vi "INTERFAZ.vi"() -> ()   [LabVIEW 2020]
panel:
  in  "Modo Nocturno":bool
  in  "stop":bool
  in  "Tab Control":enum32{"Page 1", "Page 2"}(tab)
  out "Contraseña":bool
  out "Usuario":bool
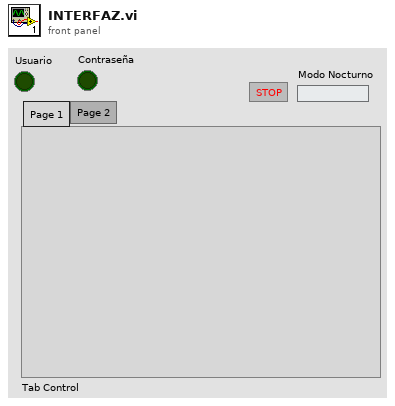
[diagram p1: front panel]
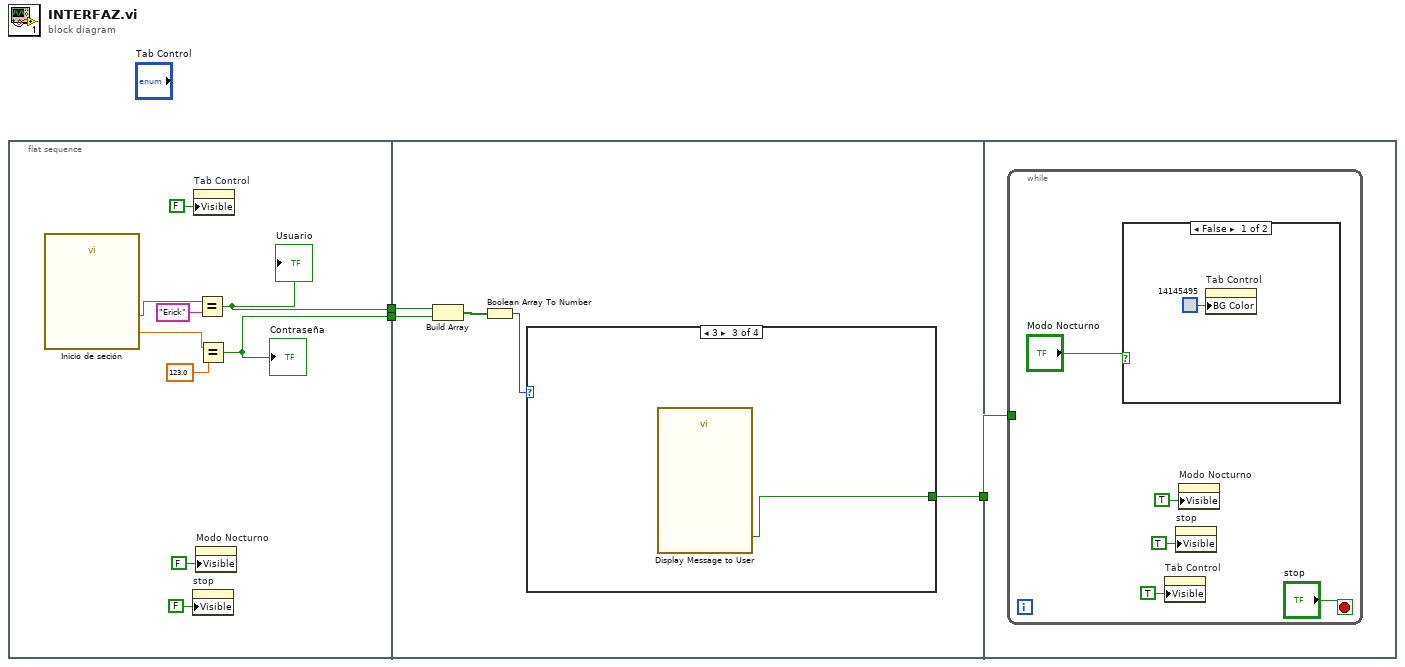
[diagram p0: block diagram]
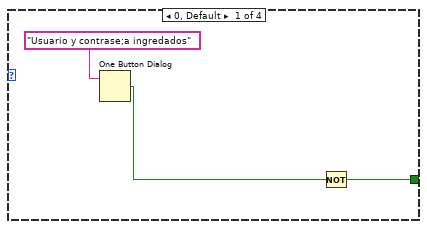
[diagram p2: hidden frame]
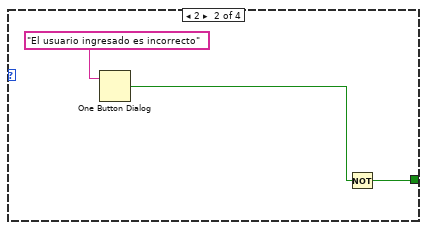
[diagram p3: hidden frame]
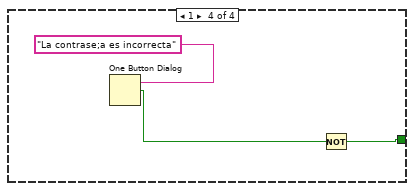
[diagram p4: hidden frame]
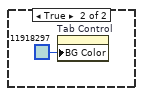
[diagram p5: hidden frame]
diagram:
  n1 = flat-sequence {
    tunnel: [w8] -> w3
    tunnel: [w7] -> w2
    tunnel: w3 -> [w17]
    tunnel: w2 -> [w16]
    tunnel: [w13] -> w1
    tunnel: w1 -> [w28]
    frame #0 {
      n2 = call "Inicio de seción"() -> ("Contraseñas"=w9:dbl, "Usuarios"=w12:string)  [unwired: 16 in, 2 out]
      n3 = property on="stop" class="Bool"("Visible"=FALSE) -> ()  [unwired: 2 in, 2 out]
      n4 = property on="Tab Control" class="TabCtl (strict)"("Visible"=FALSE) -> ()  [unwired: 2 in, 2 out]
      n5 = property on="Modo Nocturno" class="Bool (strict)"("Visible"=FALSE) -> ()  [unwired: 2 in, 2 out]
      n6 = Equal?(x=w12, y="Erick") -> (x = y?=w8:bool)
      "Usuario" <- w8
      n7 = Equal?(x=w9, y=123.0 ("Contraseñas")) -> (x = y?=w7:bool)
      "Contraseña" <- w7
    }
    frame #1 {
      n8 = Build Array(w17, w16) -> (w15:bool[])
      n9 = Boolean Array To Number(Boolean array=w15) -> (number=w14:u32)
      n10 = case shown="3" w14 {
        tunnel: [w18 w22 w24 w26] -> w13
        frame 0, Default {
          n11 = One Button Dialog(message="Usuario y contrase;a ingredados") -> (true=w19:bool)  [unwired: 1 in]
          n12 = Not(x=w19) -> (.not. x?=w18:bool)
        }
        frame 2 {
          n13 = One Button Dialog(message="El usuario ingresado es incorrecto") -> (true=w21:bool)  [unwired: 1 in]
          n14 = Not(x=w21) -> (.not. x?=w22:bool)
        }
        frame 3 {
          n15 = call "Display Message to User"() -> ("Avanzar"=w24:bool)  [unwired: 10 in, 1 out]
        }
        frame 1 {
          n16 = One Button Dialog(message="La contrase;a es incorrecta") -> (true=w25:bool)  [unwired: 1 in]
          n17 = Not(x=w25) -> (.not. x?=w26:bool)
        }
      }
    }
    frame #2 {
      n18 = while {
        tunnel: w28 -> [_]
        stop <- "stop" stop-if-true
        n19 = case shown="False" "Modo Nocturno" {
          frame False {
            n20 = property on="Tab Control" class="TabCtl (strict)"("BG Color"=u32 14145495 ("Colors:BG Color")) -> ()  [unwired: 2 in, 2 out]
          }
          frame True {
            n21 = property on="Tab Control" class="TabCtl (strict)"("BG Color"=u32 11918297 ("Colors:BG Color")) -> ()  [unwired: 2 in, 2 out]
          }
        }
        n22 = property on="Tab Control" class="TabCtl (strict)"("Visible"=TRUE) -> ()  [unwired: 2 in, 2 out]
        n23 = property on="stop" class="Bool"("Visible"=TRUE) -> ()  [unwired: 2 in, 2 out]
        n24 = property on="Modo Nocturno" class="Bool (strict)"("Visible"=TRUE) -> ()  [unwired: 2 in, 2 out]
      }
    }
  }
